vi "Write Installed Modules.vi"(8 "error in (no error)":errorcluster, 10 "Installed Modules":T1[](array[typedef]), 11 "3300 in":refnum<class "3300.lvclass">) -> (0 "error out":errorcluster, 3 "3300 out":refnum<class "3300.lvclass">)   [LabVIEW 2019, in "3300.lvlib" / "3300.lvclass"]
uses:
  Library/3300.lvclass
  Custom Controls/Modules.ctl
  Library/3300.lvclass/3300.ctl
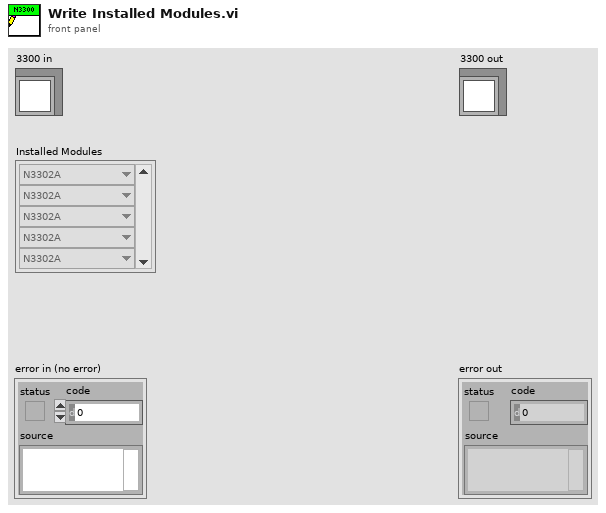
[diagram p1: front panel]
types:
  T1 = typedef "3300.lvlib/3300.lvclass/Modules.ctl" = enum16{"N3302A", "N3303A", "N3304A", "N3305A", "N3306A", "N3307A"}
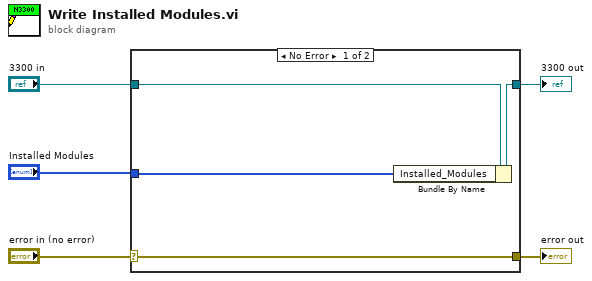
[diagram p0: block diagram]
diagram:
  n1 = case shown="No Error" "error in (no error)" {
    selector: "error in (no error)" -> [w9 w10]
    tunnel: [w9 w10] -> w4
    tunnel: [w7 w11] -> w2
    tunnel: "3300 in" -> [w8 w11]
    tunnel: "Installed Modules" -> [w6 _]
    frame No Error {
      n2 = Bundle By Name(cluster=w8, "Installed_Modules"=w6) -> (w7:refnum<class "3300.lvclass">)
    }
    frame Error {
    }
  }
  "error out" <- w4
  "3300 out" <- w2
